vi "Global Variables.vi"() -> ()   [LabVIEW 2018]
panel:
  out "SIS-10SDV502":bool
  out "SIS-10SDV501":bool
  out "SIS-10SDV500":bool
  in  "SIS-10TI101":dbl
  in  "SIS-10AI301":dbl
  in  "SIS-10LI202":dbl
  in  "SIS-10LI201":dbl
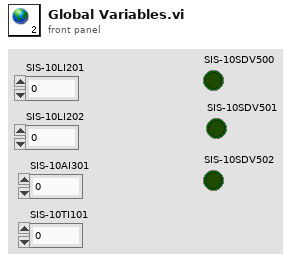
[diagram p1: front panel]
diagram:
